vi "TCP-Get Status.vi"(0 "IP Address":string, 5 "Port":i32, 11 "error in (no error)":errorcluster) -> (4 "status":bool, 15 "error out":errorcluster)   [LabVIEW 2020]
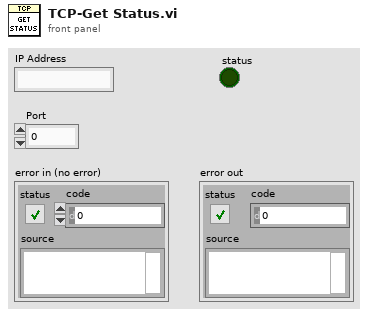
[diagram p1: front panel]
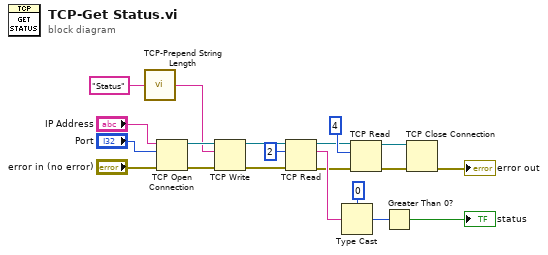
[diagram p0: block diagram]
diagram:
  n1 = call "TCP-Prepend String Length.vi"("Command"="Status" ("data string")) -> ("String"=w1:string)  [unwired: 4 in]
  n2 = TCP Open Connection(address="IP Address", remote port or service name="Port", error in (no error)="error in (no error)") -> (connection ID=w5:refnum<k5>, error out=w6:errorcluster)  [unwired: 2 in]
  n3 = TCP Write(connection ID=w5, data in=w1, error in (no error)=w6) -> (connection ID out=w4:refnum<k5>, error out=w3:errorcluster)  [unwired: 1 in, 1 out]
  n4 = TCP Read(connection ID=w4, bytes to read=2, error in (no error)=w3) -> (connection ID out=w12:refnum<k5>, data out=w13:string, error out=w11:errorcluster)  [unwired: 2 in]
  n5 = Type Cast(type=i16 0, x=w13) -> (*(type *) &x=w18:i16)
  n6 = TCP Read(connection ID=w12, bytes to read=4, error in (no error)=w11) -> (connection ID out=w17:refnum<k5>, error out=w16:errorcluster)  [unwired: 2 in, 1 out]
  n7 = Greater Than 0?(x=w18) -> (x > 0?=→"status":bool)
  n8 = TCP Close Connection(connection ID=w17, error in (no error)=w16) -> (error out=→"error out":errorcluster)  [unwired: 1 in, 1 out]
